vi "i q sum 8spc.vi"(9 "input valid":bool=TRUE, 10 "IQ in 2":T1[](array[typedef])=[{"I"=0.0, "Q"=0.0, "overflow"=FALSE}, {"I"=0.0, "Q"=0.0, "overflow"=FALSE}, {"I"=0.0, "Q"=0.0, "overflow"=FALSE}, {"I"=0.0, "Q"=0.0, "overflow"=FALSE}, {"I"=0.0, "Q"=0.0, "overflow"=FALSE}, {"I"=0.0, "Q"=0.0, "overflow"=FALSE}, {"I"=0.0, "Q"=0.0, "overflow"=FALSE}, {"I"=0.0, "Q"=0.0, "overflow"=FALSE}], 11 "IQ in":T1[](array[typedef])=[{"I"=0.0, "Q"=0.0, "overflow"=FALSE}, {"I"=0.0, "Q"=0.0, "overflow"=FALSE}, {"I"=0.0, "Q"=0.0, "overflow"=FALSE}, {"I"=0.0, "Q"=0.0, "overflow"=FALSE}, {"I"=0.0, "Q"=0.0, "overflow"=FALSE}, {"I"=0.0, "Q"=0.0, "overflow"=FALSE}, {"I"=0.0, "Q"=0.0, "overflow"=FALSE}, {"I"=0.0, "Q"=0.0, "overflow"=FALSE}]) -> (2 "output valid":bool, 3 "IQ out":T1[](array[typedef]))   [LabVIEW 2021]
doc: "sum 2 IQ datas (I+I =>I ; Q+Q =>Q ; overflow or overflow or +overflow => overflow"
uses:
  <instrlib>/_niInstr/DSP/v1/Shared/Public/IQ Data.ctl
  <instrlib>/_niInstr/DSP/v1/Shared/niInstr DSP v1 Shared.lvlib
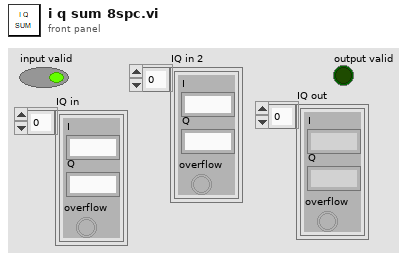
[diagram p1: front panel]
types:
  T1 = typedef "niInstr DSP v1 Shared.lvlib/IQ Data.ctl" = cluster{"I":fxp<+/-,18,1>, "Q":fxp<+/-,18,1>, "overflow":bool}
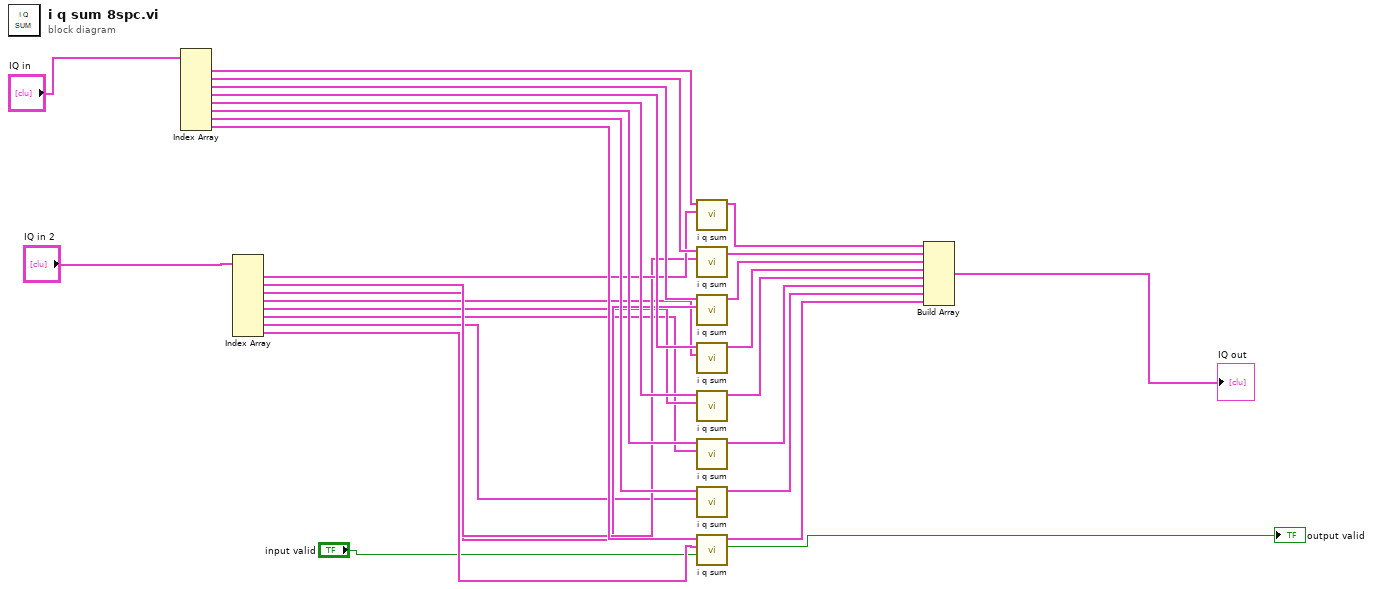
[diagram p0: block diagram]
diagram:
  n1 = Index Array(array="IQ in") -> (element #1=w27:T1, element #2=w26:T1, element #3=w25:T1, element #4=w24:T1, element #5=w23:T1, element #6=w22:T1, element #7=w21:T1, element #8=w20:T1)  [unwired: 8 in]
  n2 = Index Array(array="IQ in 2") -> (element #1=w19:T1, element #2=w18:T1, element #3=w17:T1, element #4=w16:T1, element #5=w15:T1, element #6=w14:T1, element #7=w13:T1, element #8=w12:T1)  [unwired: 8 in]
  n3 = call "i q sum.vi"(10:"data in"=w19, 11:"data in"=w27) -> ("output cluster"=w11:T1)  [unwired: 8 in, 1 out]
  n4 = call "i q sum.vi"(10:"data in"=w18, 11:"data in"=w26) -> ("output cluster"=w10:T1)  [unwired: 8 in, 1 out]
  n5 = call "i q sum.vi"(10:"data in"=w17, 11:"data in"=w25) -> ("output cluster"=w9:T1)  [unwired: 8 in, 1 out]
  n6 = call "i q sum.vi"(10:"data in"=w16, 11:"data in"=w24) -> ("output cluster"=w8:T1)  [unwired: 8 in, 1 out]
  n7 = call "i q sum.vi"(10:"data in"=w15, 11:"data in"=w23) -> ("output cluster"=w7:T1)  [unwired: 8 in, 1 out]
  n8 = call "i q sum.vi"(10:"data in"=w14, 11:"data in"=w22) -> ("output cluster"=w6:T1)  [unwired: 8 in, 1 out]
  n9 = call "i q sum.vi"(10:"data in"=w13, 11:"data in"=w21) -> ("output cluster"=w5:T1)  [unwired: 8 in, 1 out]
  n10 = call "i q sum.vi"("input valid"="input valid", 10:"data in"=w12, 11:"data in"=w20) -> ("output valid"=→"output valid":bool, "output cluster"=w4:T1)  [unwired: 7 in]
  n11 = Build Array(w11, w10, w9, w8, w7, w6, w5, w4) -> (→"IQ out":T1[])
